vi "Query Capabilities (Current).vi"(0 "VISA resource name":refnum<visa-resource-name>, 5 "Absolute Maximums (T)":bool=TRUE, 11 "error in (no error)":errorcluster) -> (4 "VISA resource name out":refnum<visa-resource-name>, 6 "Current Capabilities":T1, 15 "error out":errorcluster)   [LabVIEW 2020, in "NH Research Regenerative Test Series.lvlib"]
doc: "Returns various Current capabilities of the module."
uses:
  NH Research Regenerative Test Series.lvlib
  Current Capabilities.ctl
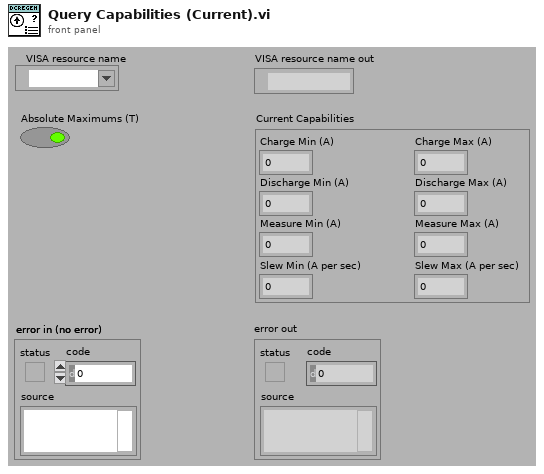
[diagram p1: front panel]
types:
  T1 = typedef "NH Research Regenerative Test Series.lvlib/Current Capabilities.ctl" = cluster{"Charge Min (A)":dbl, "Charge Max (A)":dbl, "Discharge Min (A)":dbl, "Discharge Max (A)":dbl, "Measure Min (A)":dbl, "Measure Max (A)":dbl, "Slew Min (A per sec)":dbl, "Slew Max (A per sec)":dbl}
  T2 = cluster{"[0]":dbl, "[1]":dbl, "[2]":dbl, "[3]":dbl, "[4]":dbl, "[5]":dbl, "[6]":dbl, "[7]":dbl}
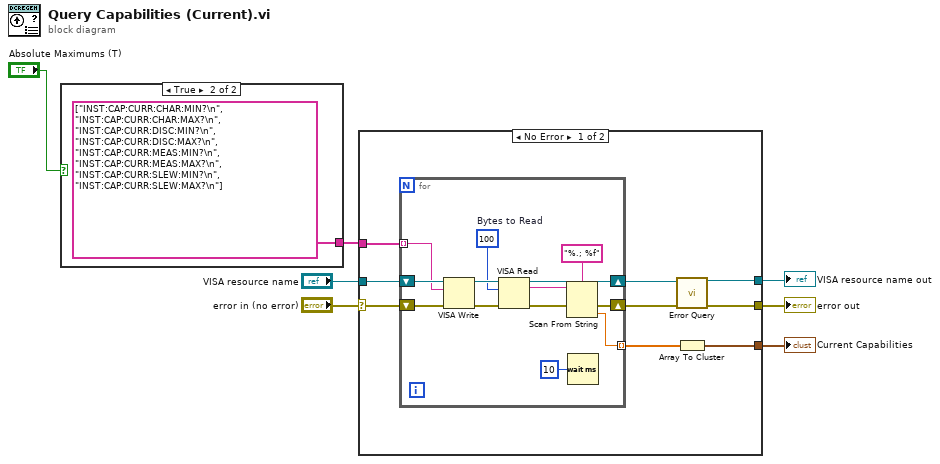
[diagram p0: block diagram]
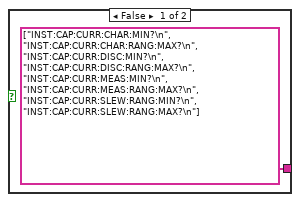
[diagram p2: hidden frame]
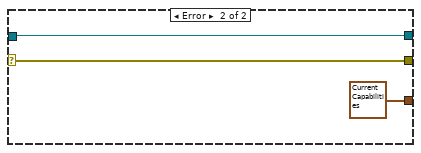
[diagram p3: hidden frame]
diagram:
  n1 = case shown="True" "Absolute Maximums (T)" {
    tunnel: [string[] ["INST:CAP:CURR:CHAR:MIN?\n", "INST:CAP:CURR:CHAR:RANG:MAX?\n", "INST:CAP:CURR:DISC:MIN?\n", "INST:CAP:CURR:DISC:RANG:MAX?\n", "INST:CAP:CURR:MEAS:MIN?\n", "INST:CAP:CURR:MEAS:RANG:MAX?\n", "INST:CAP:CURR:SLEW:RANG:MIN?\n", "INST:CAP:CURR:SLEW:RANG:MAX?\n"] string[] ["INST:CAP:CURR:CHAR:MIN?\n", "INST:CAP:CURR:CHAR:MAX?\n", "INST:CAP:CURR:DISC:MIN?\n", "INST:CAP:CURR:DISC:MAX?\n", "INST:CAP:CURR:MEAS:MIN?\n", "INST:CAP:CURR:MEAS:MAX?\n", "INST:CAP:CURR:SLEW:MIN?\n", "INST:CAP:CURR:SLEW:MAX?\n"]] -> w3
    frame False {
    }
    frame True {
    }
  }
  n2 = case shown="No Error" "error in (no error)" {
    selector: "error in (no error)" -> [w17 w34]
    tunnel: [w12 w34] -> w6
    tunnel: [w18 w33] -> w4
    tunnel: "VISA resource name" -> [w16 w33]
    tunnel: w3 -> [w15 _]
    tunnel: [w11 T1 {"Charge Min (A)"=nan, "Charge Max (A)"=nan, "Discharge Min (A)"=nan, "Discharge Max (A)"=nan, "Measure Min (A)"=nan, "Measure Max (A)"=nan, "Slew Min (A per sec)"=nan, "Slew Max (A per sec)"=nan}] -> w2
    frame No Error {
      n3 = for {
        tunnel: w15 -> [w26] mode=indexing
        tunnel: [w22] -> w14 mode=indexing
        shift-right: [w21] -> w13
        shift-left: w17 -> [w28]
        shift-right: [w20] -> w10
        shift-left: w16 -> [w27]
        w29 = u32 100  # Bytes to Read
        n4 = VISA Write(VISA resource name=w27, write buffer=w26, error in (no error)=w28) -> (VISA resource name out=w30:refnum<visa-resource-name>, error out=w31:errorcluster)  [unwired: 1 out]
        n5 = VISA Read(VISA resource name=w30, byte count=w29, error in (no error)=w31) -> (VISA resource name out=w20:refnum<visa-resource-name>, read buffer=w23:string, error out=w24:errorcluster)  [unwired: 1 out]
        n6 = Scan From String(format string="%.; %f", input string=w23, error in=w24) -> (error out=w21:errorcluster, output 1=w22:dbl)  [unwired: 2 in, 2 out]
        n7 = Wait (ms)(milliseconds to wait=u32 10) -> ()  [unwired: 1 out]
      }
      n8 = call "Error Query.vi"("VISA resource name"=w10, "error in (no error)"=w13) -> ("VISA resource name out"=w18:refnum<visa-resource-name>, "error out"=w12:errorcluster)  [unwired: 10 in, 2 out]
      n9 = Array To Cluster(array=w14) -> (cluster=w11:T2)
    }
    frame Error {
    }
  }
  "error out" <- w6
  "VISA resource name out" <- w4
  "Current Capabilities" <- w2
